vi "Apply selectors to all GObjects on a panel.vi"(8 "Error in":errorcluster, 11 "VI in":refnum<vi>) -> (0 "Error out":errorcluster, 3 "Elapsed time":dbl)   [LabVIEW 2019, in "LSS.lvlib"]
uses:
  LSS.lvlib
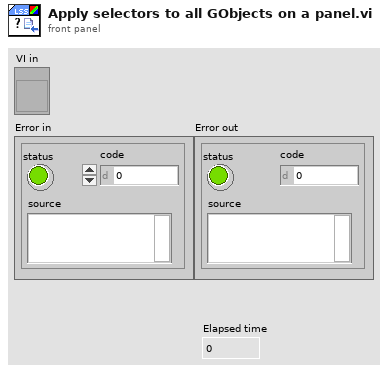
[diagram p1: front panel]
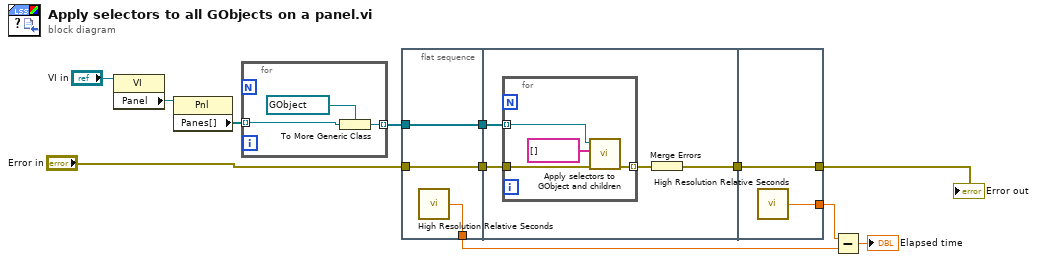
[diagram p0: block diagram]
diagram:
  n1 = property class="VI"(reference="VI in") -> ("Panel"=w3:refnum<vi>)  [unwired: 1 in, 2 out]
  n2 = property class="Pnl"(reference=w3) -> ("Panes[]"=w4:refnum<vi>[])  [unwired: 1 in, 2 out]
  n3 = for {
    tunnel: w4 -> [w15] mode=indexing
    tunnel: [w14] -> w5 mode=indexing
    n4 = To More Generic Class(target class=refnum<vi> refnum, reference=w15) -> (generic class reference=w14:refnum<vi>)
  }
  n5 = flat-sequence {
    tunnel: "Error in" -> [w17]
    tunnel: w5 -> [w18]
    tunnel: [w18] -> w12
    tunnel: [w17] -> w11
    tunnel: [w16] -> w8
    tunnel: w12 -> [w22]
    tunnel: w11 -> [w21]
    tunnel: [w19] -> w10
    tunnel: [w28] -> w7
    tunnel: [w27] -> w9
    tunnel: w10 -> [w27]
    frame #0 {
      n6 = call <vilib>:"High Resolution Relative Seconds.vi"() -> ("relative seconds"=w16:dbl)
    }
    frame #1 {
      n7 = for {
        tunnel: w22 -> [w26] mode=indexing
        tunnel: w21 -> [w24]
        tunnel: [w23] -> w20 mode=indexing
        n8 = call "Apply selectors to GObject and children.vi"("Error in"=w24, "Owning item selectors"=string[] [], "GObject in"=w26) -> ("Error out"=w23:errorcluster)  [unwired: 8 in]
      }
      n9 = Merge Errors(w20) -> (w19:errorcluster)
    }
    frame #2 {
      n10 = call <vilib>:"High Resolution Relative Seconds.vi"() -> ("relative seconds"=w28:dbl)
    }
  }
  n11 = Subtract(x=w7, y=w8) -> (x-y=→"Elapsed time":dbl)
  "Error out" <- w9
